vi "Indicators.vi"() -> ()   [LabVIEW 2019]
panel:
  out "Thermometer":dbl(slide) scale=0.0..100.0
  out "String 2":string
  out "Boolean 2":bool
  out "Numeric 2":dbl
  in  "String":string
  in  "Boolean":bool
  in  "Set Temp":dbl(slide) scale=0.0..100.0
  in  "Numeric":dbl
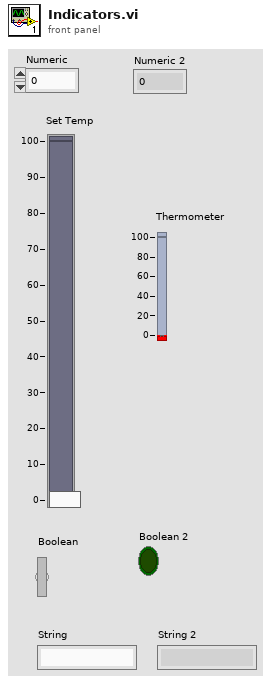
[diagram p1: front panel]
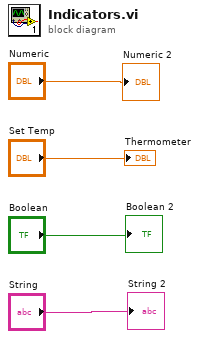
[diagram p0: block diagram]
diagram:
  "Numeric 2" <- "Numeric"
  "Boolean 2" <- "Boolean"
  "String 2" <- "String"
  "Thermometer" <- "Set Temp"
